vi "capstone1 ver 4_temp&move code.vi"() -> ()   [LabVIEW 2016]
uses:
  <instrlib>/Dynamixel Motor/Public/Motor Operation/Low Level/Baud Setting.ctl
  <vilib>/myRIO/Instrument Drivers/Onboard IO/DIO/typedefs/DIO Reference.ctl
  <vilib>/myRIO/Common/Instrument Driver Framework/Utilities/typedefs/myRIO Generic Hardware Reference.ctl
  <vilib>/myRIO/Common/Instrument Driver Framework/Utilities/typedefs/Hardware Version Enum.ctl
  <vilib>/myRIO/Common/Instrument Driver Framework/Utilities/typedefs/myRIO v1.0 Reference.ctl
  <vilib>/myRIO/Common/Instrument Driver Framework/Utilities/typedefs/Generic FPGA Reference.ctl
  <vilib>/myRIO/Common/Instrument Driver Framework/myRIO v1.0/DIO/typedefs/DIO Channels List.ctl
  <vilib>/myRIO/Common/Instrument Driver Framework/myRIO v1.0/DIO/typedefs/DIO Channels Enum.ctl
  <vilib>/userdefined/High Color/nirio_resource_hc.ctl
  <vilib>/myRIO/Common/Instrument Driver Framework/Utilities/vis/Is FPGA Ref Available.vi
  <vilib>/myRIO/Common/Instrument Driver Framework/myRIO v1.0/DIO/vis/myRIO v1.1 Open DIO.vi
  <vilib>/myRIO/Instrument Drivers/Onboard IO/DIO/vis/Write.vi
  <vilib>/myRIO/Common/Instrument Driver Framework/Utilities/vis/Validate Channels.vi
  <vilib>/myRIO/Common/Instrument Driver Framework/myRIO v1.0/DIO/vis/myRIO v1.0 Reserve DIO.vi
  <vilib>/myRIO/Common/Instrument Driver Framework/myRIO v1.0/Resource Manager/vis/myRIO v1.0 Reserve Channel List.vi
  <vilib>/myRIO/Common/Instrument Driver Framework/myRIO v1.0/DIO/vis/myRIO v1.0 Build MUX Configuration DIO.vi
  <vilib>/myRIO/Common/Instrument Driver Framework/myRIO v1.0/Resource Manager/vis/myRIO v1.0 Reserve Channel.vi
  <vilib>/myRIO/Common/Instrument Driver Framework/myRIO v1.0/Resource Manager/vis/myRIO v1.0 Unreserve Channel.vi
  <vilib>/myRIO/Common/Instrument Driver Framework/myRIO v1.0/Resource Manager/vis/myRIO v1.0 Create Configuration List.vi
  <vilib>/myRIO/Common/Instrument Driver Framework/myRIO v1.0/Resource Manager/vis/myRIO v1.0 Build Mutex Name.vi
  <vilib>/Utility/VariantDataType/GetNumericInfo.vi
  <vilib>/Utility/error.llb/Error Cluster From Error Code.vi
  <vilib>/myRIO/Common/Instrument Driver Framework/myRIO v1.0/myRIO v1.1 Open.vi
  <vilib>/myRIO/Common/Instrument Driver Framework/Utilities/vis/IO Manager.vi
  <vilib>/myRIO/Common/Instrument Driver Framework/Utilities/vis/Configuration Manager.vi
  <vilib>/myRIO/Common/Instrument Driver Framework/myRIO v1.0/Resource Manager/vis/myRIO v1.0 Configure IO.vi
  <vilib>/myRIO/Common/Instrument Driver Framework/myRIO v1.0/myRIO v1.0 Close.vi
  <vilib>/myRIO/Common/Instrument Driver Framework/myRIO v1.0/DIO/vis/myRIO v1.0 Write DIO.vi
  <vilib>/myRIO/Express VI/Onboard Devices/LED/LED Express VI.xnode
  <vilib>/myRIO/Instrument Drivers/Onboard IO/DIO/vis/myRIO DIO Open.xnode
  <instrlib>/Dynamixel Motor/Dynamixel Motor.lvlib
  <vilib>/myRIO/Instrument Drivers/Onboard IO/DIO/DIO.lvlib
panel:
  out "RT TCP Loop time 4":u32
  out "Numeric":i32
  out "RT TCP Loop time 3":u32
  out "RT TCP Loop time 2":u32
  out "RT TCP Loop time":u32
  out "motor temp":cluster{"0":sgl, "1":sgl, "2":sgl, "3":sgl}
  out "value":T1
  out "TCP Read data":string
  in  "정지":bool
  out "error out":errorcluster
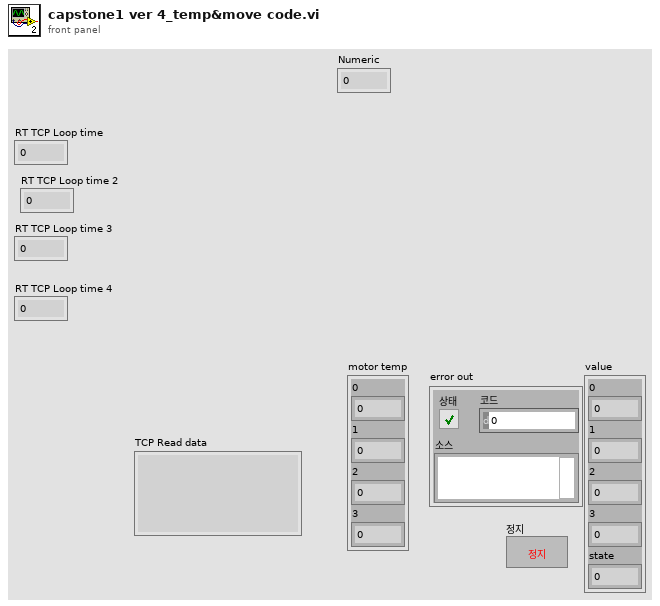
[diagram p1: front panel]
types:
  T1 = cluster{"0":sgl, "1":sgl, "2":sgl, "3":sgl, "state":sgl}
  T2 = typedef "Dynamixel Motor.lvlib/Baud Setting.ctl" = u8
  T3 = enum16{"big-endian, network order", "native, host order", "little-endian"}
  T4 = typedef "DIO.lvlib/DIO Reference.ctl" = cluster{"myRIO Reference":T5, "DIO Channels List":T9}
  T5 = typedef "myRIO Generic Hardware Reference.ctl" = cluster{"myRIO Model":T6, "myRIO Hardware Reference":T7}
  T6 = typedef "Hardware Version Enum.ctl" = enum16{"Unknown", "myRIO-1900", "myRIO-1950", "roboRIO", "NI ELVIS RIO CM"}
  T7 = typedef "myRIO v1.0 Reference.ctl" = cluster{"Generic FPGA Reference":T8, "Allow multiple opens":bool}
  T8 = typedef "Generic FPGA Reference.ctl" = refnum<k20>
  T9 = typedef "DIO Channels List.ctl" = T10[]
  T10 = typedef "DIO Channels Enum.ctl" = enum16{"Not Connected", "C/DIO0", "C/DIO1", "C/DIO2", "C/DIO3", "C/DIO4", "C/DIO5", "C/DIO6", "C/DIO7", "A/DIO0", "A/DIO1", "A/DIO2", "A/DIO3", "A/DIO4", "A/DIO5", "A/DIO6", "A/DIO7", "A/DIO8", "A/DIO9", "A/DIO10", "A/DIO11", "A/DIO12", "A/DIO13", "A/DIO14", "A/DIO15", "B/DIO0", "B/DIO1", "B/DIO2", "B/DIO3", "B/DIO4", "B/DIO5", "B/DIO6", "B/DIO7", "B/DIO8", "B/DIO9", "B/DIO10", "B/DIO11", "B/DIO12", "B/DIO13", "B/DIO14", "B/DIO15", "LED0", "LED1", "LED2", "LED3", "Button0", "DIO/DIO0", "DIO/DIO1", "DIO/DIO2", "DIO/DIO3", "DIO/DIO4", "DIO/DIO5", "DIO/DIO6", "DIO/DIO7", "DIO/DIO8", "DIO/DIO9", "SPI/CS0", "SPI/CS1", "SPI/CS2", "SPI/CS3", "LED RADIO (Green)", "LED RADIO (Red)", "LED COMM (Green)", "LED COMM (Red)", "LED MODE (Green)", "LED MODE (Red)"}
  T11 = typedef "nirio_resource_hc.ctl" = tag
  T12 = cluster{"0":sgl, "1":sgl, "2":sgl, "3":sgl, "state":i32}
  T13 = cluster{"Temperature (C)":u8, "Temperature (C)":u8, "Temperature (C)":u8, "Temperature (C)":u8}
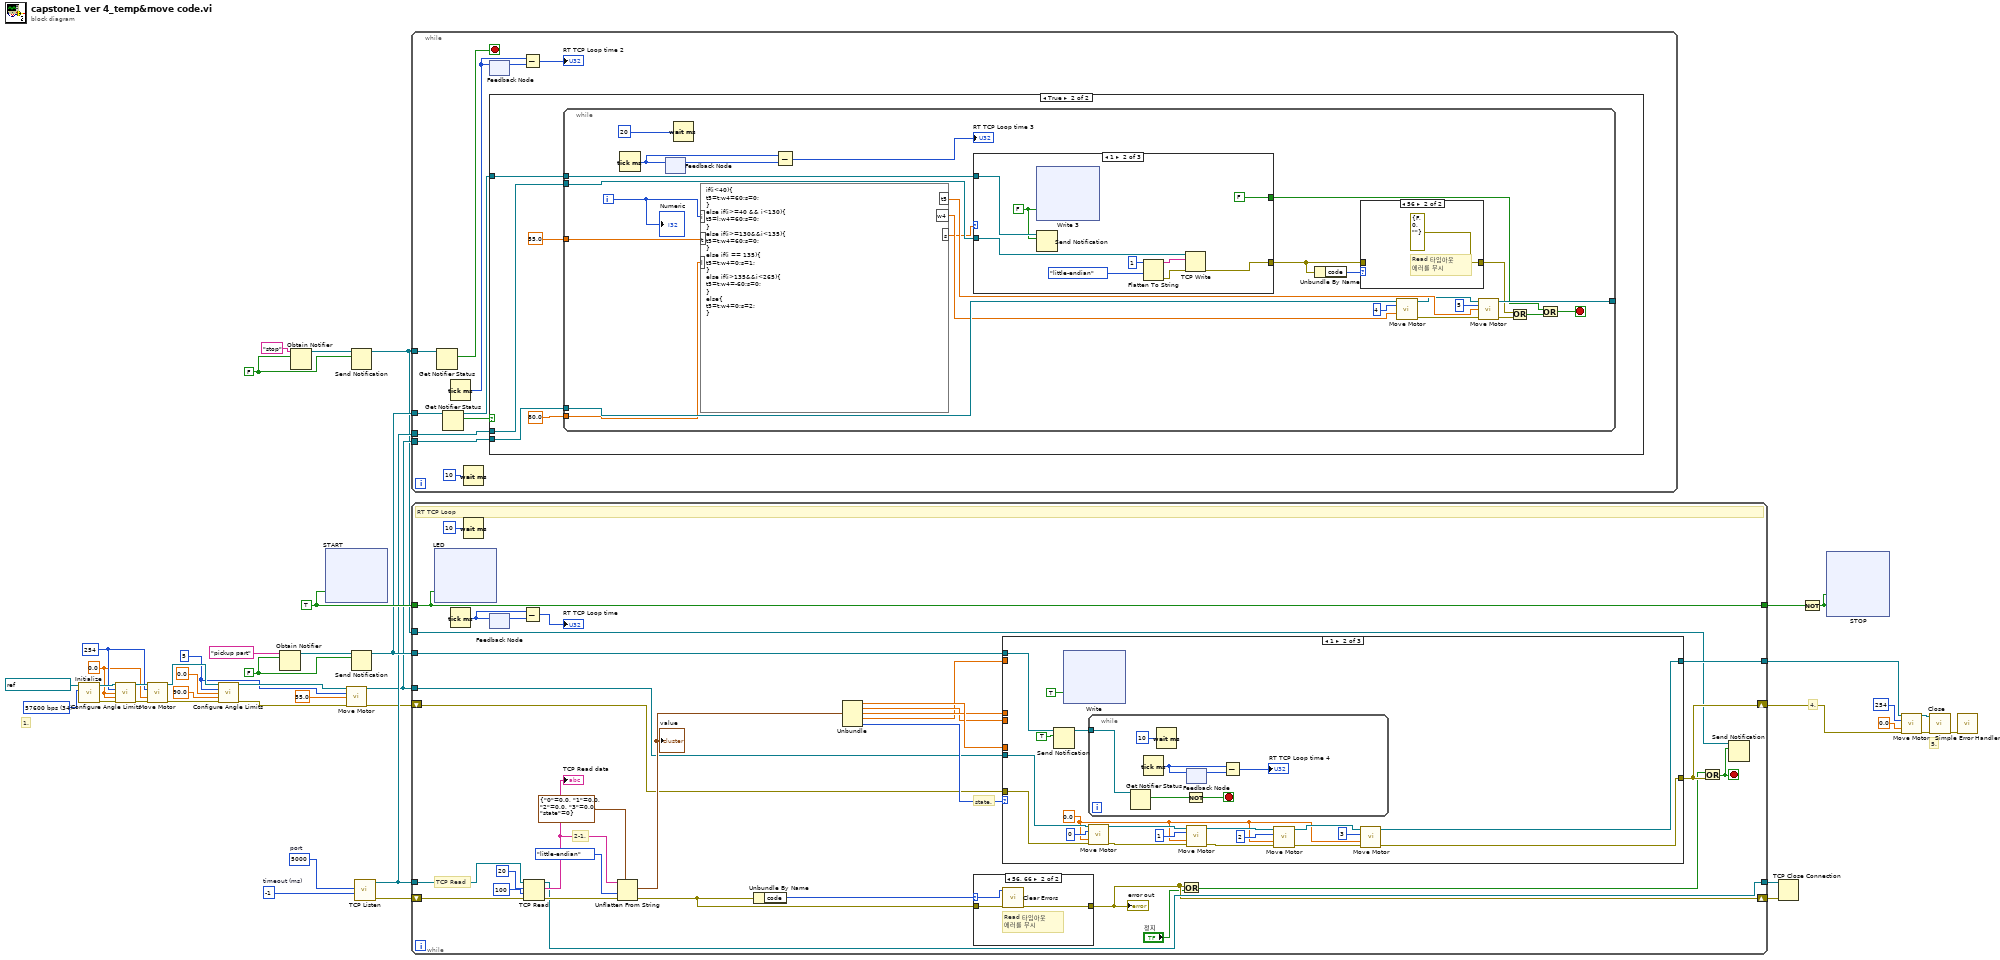
[diagram p0: block diagram]
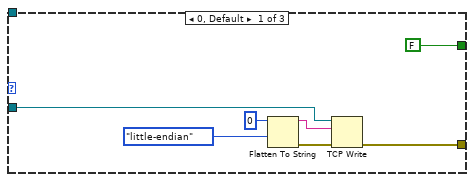
[diagram p4: hidden frame]
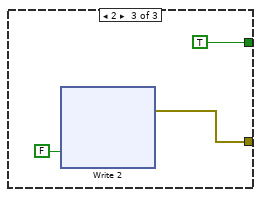
[diagram p5: hidden frame]
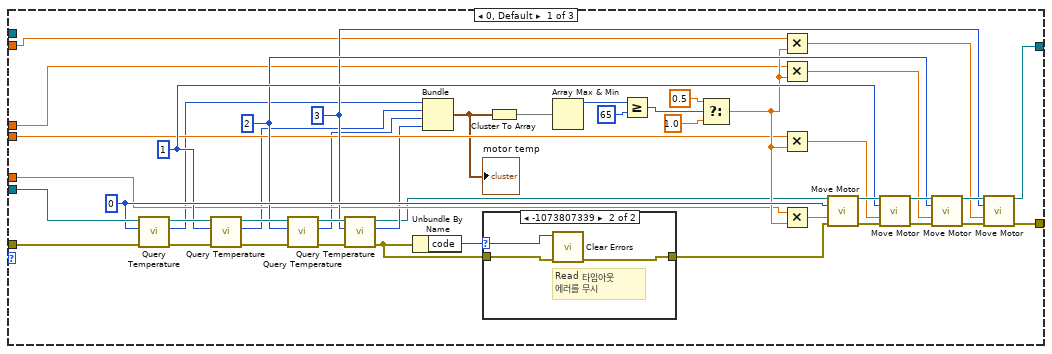
[diagram p6: hidden frame]
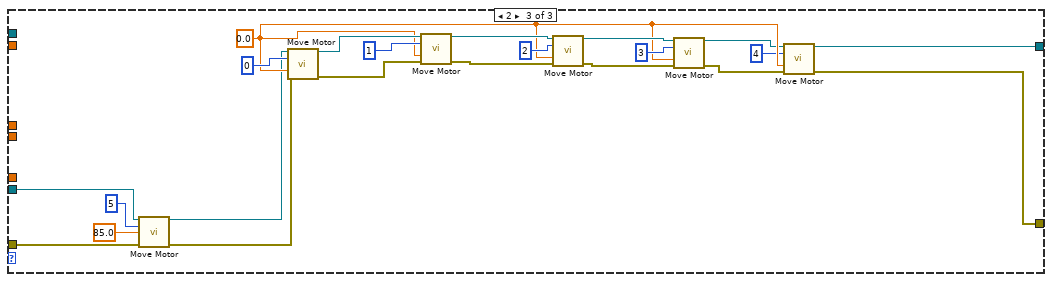
[diagram p8: hidden frame]
diagram:
  w3 = FALSE
  w14 = FALSE
  w6 = 5
  w37 = T2 34 items=["1,000,000 bps"=1, "500,000 bps"=3, "400,000 bps"=4, "250,000 bps"=7, "200,000 bps"=9, "115200 bps"=16, "57600 bps"=34, "19200 bps"=103, "9600 bps"=207] ("Baud rate (57600 bps)")
  w22 = TRUE
  w24 = u8 254 ("Motor ID (0)")
  w23 = 0.0 ("Clockwise Angle Limit (0 deg)")
  w41 = u16 5000  # port
  w42 = -1  # timeout (ms)
  # "5."
  # "4."
  # "1."
  n1 = call <instrlib>:"Initialize.vi"("Baud rate (57600 bps)"=w37, "VISA resource name"=refnum<visa-resource-name> "ASRL3::INSTR") -> ("error out"=w31:errorcluster, "VISA resource name out"=w30:refnum<visa-resource-name>)  [unwired: 8 in]
  n2 = call <instrlib>:"Configure Angle Limits.vi"("VISA resource name"=w30, "Motor ID (0)"=w24, "Clockwise Angle Limit (0 deg)"=w23, "Counter-Clockwise Angle Limit (300 deg)"=w23, "error in (no error)"=w31) -> ("VISA resource name out"=w26:refnum<visa-resource-name>, "error out"=w25:errorcluster)  [unwired: 9 in]
  n3 = call <instrlib>:"Move Motor.vi"("VISA resource name"=w26, "Motor ID (0)"=w24, "Goal Speed (RPM)"=w23, "error in (no error)"=w25) -> ("VISA resource name out"=w20:refnum<visa-resource-name>, "error out"=w21:errorcluster)  [unwired: 10 in]
  n4 = call <instrlib>:"Configure Angle Limits.vi"("VISA resource name"=w20, "Motor ID (0)"=w6, "Clockwise Angle Limit (0 deg)"=0.0, "Counter-Clockwise Angle Limit (300 deg)"=90.0 ("Clockwise Angle Limit (0 deg)"), "error in (no error)"=w21) -> ("VISA resource name out"=w10:refnum<visa-resource-name>, "error out"=w9:errorcluster)  [unwired: 9 in]
  n5 = Obtain Notifier(name (unnamed)="pickup part", notification data type=w14) -> (notifier out=w15:refnum<notifier>)  [unwired: 2 in, 2 out]
  n6 = Obtain Notifier(name (unnamed)="stop", notification data type=w3) -> (notifier out=w4:refnum<notifier>)  [unwired: 2 in, 2 out]
  n7 = xnode "START"("LED0"=w22) -> ()  [unwired: 1 in, 1 out]
  n8 = call <instrlib>:"Move Motor.vi"("VISA resource name"=w10, "Motor ID (0)"=w6, "Goal Position (180 deg)"=55.0, "error in (no error)"=w9) -> ("VISA resource name out"=w7:refnum<visa-resource-name>, "error out"=w8:errorcluster)  [unwired: 10 in]
  n9 = Send Notification(notification=w3, notifier=w4) -> (notifier out=w1:refnum<notifier>)  [unwired: 1 in, 1 out]
  n10 = Send Notification(notification=w14, notifier=w15) -> (notifier out=w13:refnum<notifier>)  [unwired: 1 in, 1 out]
  n11 = call <vilib>:"TCP Listen.vi"("timeout ms (wait forever: -1)"=w42, "port"=w41) -> ("error out"=w38:errorcluster, "connection ID"=w12:refnum<k5>)  [unwired: 5 in, 3 out]
  n12 = while {
    tunnel: w13 -> [w52]
    tunnel: w7 -> [w49]
    tunnel: w12 -> [w48]
    tunnel: w1 -> [w44]
    stop <- w43 stop-if-true
    n13 = Get Notifier Status(notifier=w44) -> (current notification=w43:bool)  [unwired: 1 in, 4 out]
    n14 = Get Notifier Status(notifier=w52) -> (notifier out=w50:refnum<notifier>, current notification=w51:bool)  [unwired: 1 in, 3 out]
    n15 = Tick Count (ms)() -> (millisecond timer value=w46:u32)
    n16 = Wait (ms)(milliseconds to wait=u32 10 ("대기 시간 (ms)")) -> ()  [unwired: 1 out]
    n17 = feedback #1() -> (w47:u32)  [unwired: 1 in]
    n18 = feedback-in #1(w46) -> ()
    n19 = case shown="True" w51 {
      tunnel: w50 -> [_ w54]
      tunnel: w49 -> [_ w58]
      tunnel: w48 -> [_ w57]
      frame False {
      }
      frame True {
        n20 = while {
          tunnel: w57 -> [w78]
          tunnel: w58 -> [w82]
          tunnel: [w77] -> _
          tunnel: 55.0 -> [w74]
          tunnel: 80.0 -> [w73]
          tunnel: w54 -> [w71]
          i -> [w80]
          stop <- w62 stop-if-true
          n21 = Tick Count (ms)() -> (millisecond timer value=w68:u32)
          n22 = feedback #2() -> (w69:u32)  [unwired: 1 in]
          n23 = feedback-in #2(w68) -> ()
          n24 = Wait (ms)(milliseconds to wait=u32 20 ("대기 시간 (ms)")) -> ()  [unwired: 1 out]
          n25 = formula code="if(i<40){\nt5=t;w4=60;s=0;\n}\nelse if(i>=40 && i<130){\nt5=l;w4=60;s=0;\n}\nelse if(i>=130&&i<135){\nt5=t;w4=60;s=0;\n}\nelse if(i == 135){\nt5=t;w4=0;s=1;\n}\nelse if(i>135&&i<265){\nt5=t;w4=-60;s=0;\n}\nelse{\nt5=t;w4=0;s=2;\n}"("i"=w80, "t"=w74, "l"=w73) -> ("t5"=w75:dbl, "w4"=w79:dbl, "s"=w70:dbl)
          n26 = Subtract(x=w68, y=w69) -> (x-y=→"RT TCP Loop time 3":u32)
          n27 = case shown="1" w70 {
            tunnel: w78 -> [w89 w101 _]
            tunnel: w71 -> [_ w97 _]
            tunnel: [FALSE FALSE TRUE] -> w64
            tunnel: [w86 w94 w137] -> w60
            frame 0, Default {
              n28 = Flatten To String(anything=0, byte order (0:big-endian, network order)=T3."little-endian") -> (data string=w90:string, error out=w87:errorcluster)  [unwired: 2 in, 1 out]
              n29 = TCP Write(connection ID=w89, data in=w90, error in (no error)=w87) -> (error out=w86:errorcluster)  [unwired: 1 in, 2 out]
            }
            frame 1 {
              w93 = FALSE ("notification")
              n30 = xnode "Write 3"("LED2"=w93) -> ()  [unwired: 1 in, 1 out]
              n31 = Send Notification(notification=w93, notifier=w97) -> ()  [unwired: 1 in, 2 out]
              n32 = Flatten To String(anything=1, byte order (0:big-endian, network order)=T3."little-endian") -> (data string=w98:string, error out=w95:errorcluster)  [unwired: 2 in, 1 out]
              n33 = TCP Write(connection ID=w101, data in=w98, error in (no error)=w95) -> (error out=w94:errorcluster)  [unwired: 1 in, 2 out]
            }
            frame 2 {
              n34 = xnode "Write 2"("LED2"=FALSE) -> ("error out"=w137:errorcluster)  [unwired: 1 in]
            }
          }
          n35 = Unbundle By Name(w60) -> ("code"=w61:i32)
          n36 = case shown="56" w61 {
            tunnel: [w84 errorcluster {"status"=FALSE, "code"=0, "source"=""} ("에러 출력")] -> w59
            tunnel: w60 -> [w84 _]
            frame 0, Default {
            }
            frame 56 {
              # "Read 타임아웃\n에러를 무시"
            }
          }
          n37 = call <instrlib>:"Move Motor.vi"("VISA resource name"=w82, "Motor ID (0)"=4, "Goal Speed (RPM)"=w79) -> ("VISA resource name out"=w72:refnum<visa-resource-name>, "error out"=w66:errorcluster)  [unwired: 11 in]
          n38 = call <instrlib>:"Move Motor.vi"("VISA resource name"=w72, "Motor ID (0)"=5, "Goal Position (180 deg)"=w75, "error in (no error)"=w66) -> ("VISA resource name out"=w77:refnum<visa-resource-name>, "error out"=w65:errorcluster)  [unwired: 10 in]
          n39 = Or(x=w59, y=w65) -> (x .or. y?=w63:bool)
          n40 = Or(x=w64, y=w63) -> (x .or. y?=w62:bool)
          "Numeric" <- w80
        }
      }
    }
    n41 = Subtract(x=w46, y=w47) -> (x-y=→"RT TCP Loop time 2":u32)
  }
  n42 = while {
    tunnel: w12 -> [w196]
    tunnel: [w180] -> w40
    shift-right: [w179] -> w39
    shift-left: w38 -> [w197]
    shift-right: [w186] -> w19
    shift-left: w8 -> [w185]
    tunnel: w22 -> [w195]
    tunnel: [w195] -> w33
    tunnel: w7 -> [w188]
    tunnel: [w187] -> w18
    tunnel: w13 -> [w178]
    tunnel: w1 -> [w176]
    stop <- w175 stop-if-true
    # "state."
    # "2-1."
    # "TCP Read"
    # "RT TCP Loop"
    n43 = xnode "LED"("LED1"=w195) -> ()  [unwired: 1 in, 1 out]
    n44 = Tick Count (ms)() -> (millisecond timer value=w182:u32)
    n45 = Wait (ms)(milliseconds to wait=u32 10 ("대기 시간 (ms)")) -> ()  [unwired: 1 out]
    n46 = feedback #3() -> (w183:u32)  [unwired: 1 in]
    n47 = feedback-in #3(w182) -> ()
    n48 = Subtract(x=w182, y=w183) -> (x-y=→"RT TCP Loop time":u32)
    n49 = TCP Read(connection ID=w196, bytes to read=20 ("읽을 바이트"), error in (no error)=w197, 9:100 ("타임아웃 ms (25000)")) -> (connection ID out=w180:refnum<k5>, data out=w200:string, error out=w199:errorcluster)  [unwired: 1 in]
    "TCP Read data" <- w200
    n50 = Unflatten From String(type=T12 {"0"=0.0, "1"=0.0, "2"=0.0, "3"=0.0, "state"=0}, binary string=w200, byte order (0:big-endian, network order)=T3."little-endian", error in (no error)=w199) -> (value=w194:T12, error out=w198:errorcluster)  [unwired: 1 in, 1 out]
    "value" <- w194
    n51 = Unbundle By Name(w198) -> ("code"=w205:i32)
    n52 = Unbundle(w194) -> ("0"=w193:sgl, "1"=w191:sgl, "2"=w192:sgl, "3"=w190:sgl, "state"=w189:i32)
    n53 = case shown="56, 66" w205 {
      selector: w205 -> [_ w375]
      tunnel: [w373 w374] -> w179
      tunnel: w198 -> [w373 w376]
      frame 0, Default {
      }
      frame 56, 66 {
        # "Read 타임아웃\n에러를 무시"
        n54 = call <vilib>:"Clear Errors.vi"("error in (no error)"=w376, "specific error code to clear (0: all)"=w375) -> ("error out"=w374:errorcluster)  [unwired: 4 in, 1 out]
      }
    }
    "error out" <- w179
    n55 = case shown="1" w189 {
      tunnel: w193 -> [w229 _ _]
      tunnel: w191 -> [w227 _ _]
      tunnel: w192 -> [w225 _ _]
      tunnel: w190 -> [w223 _ _]
      tunnel: w188 -> [w241 w263 w318]
      tunnel: [w211 w260 w324] -> w187
      tunnel: [w212 w259 w323] -> w186
      tunnel: w185 -> [w213 w261 w320]
      tunnel: w178 -> [_ w258 _]
      frame 0, Default {
        w237 = 3
        w238 = 2
        w239 = 1
        w240 = 0
        n56 = call <instrlib>:"Query Temperature.vi"("error in"=w213, "Motor ID (0)"=w240, "VISA resource name"=w241) -> ("error out"=w236:errorcluster, "Temperature (C)"=w221:u8, "VISA resource name out"=w244:refnum<visa-resource-name>)  [unwired: 6 in]
        n57 = call <instrlib>:"Query Temperature.vi"("error in"=w236, "Motor ID (0)"=w239, "VISA resource name"=w244) -> ("error out"=w235:errorcluster, "Temperature (C)"=w220:u8, "VISA resource name out"=w243:refnum<visa-resource-name>)  [unwired: 6 in]
        n58 = call <instrlib>:"Query Temperature.vi"("error in"=w235, "Motor ID (0)"=w238, "VISA resource name"=w243) -> ("error out"=w234:errorcluster, "Temperature (C)"=w219:u8, "VISA resource name out"=w242:refnum<visa-resource-name>)  [unwired: 6 in]
        n59 = call <instrlib>:"Query Temperature.vi"("error in"=w234, "Motor ID (0)"=w237, "VISA resource name"=w242) -> ("error out"=w208:errorcluster, "Temperature (C)"=w218:u8, "VISA resource name out"=w210:refnum<visa-resource-name>)  [unwired: 6 in]
        n60 = Unbundle By Name(w208) -> ("code"=w209:i32)
        n61 = Bundle("Temperature (C)"=w221, "Temperature (C)"=w220, "Temperature (C)"=w219, "Temperature (C)"=w218) -> (w215:T13)  [unwired: 1 in]
        "motor temp" <- w215
        n62 = case shown="-1073807339" w209 {
          selector: w209 -> [_ w253]
          tunnel: [w251 w252] -> w207
          tunnel: w208 -> [w251 w254]
          frame 0, Default {
          }
          frame -1073807339 {
            # "Read 타임아웃\n에러를 무시"
            n63 = call <vilib>:"Clear Errors.vi"("error in (no error)"=w254, "specific error code to clear (0: all)"=w253) -> ("error out"=w252:errorcluster)  [unwired: 4 in, 1 out]
          }
        }
        n64 = Cluster To Array(cluster=w215) -> (array=w217:u8[])
        n65 = Array Max & Min(array=w217) -> (max value=w216:u8)  [unwired: 3 out]
        n66 = Greater Or Equal?(x=w216, y=65) -> (x >= y?=w214:bool)
        n67 = Select(t=0.5, s=w214, f=1.0) -> (s? t:f=w230:dbl)
        n68 = Multiply(x=w223, y=w230) -> (x*y=w222:dbl)
        n69 = Multiply(x=w225, y=w230) -> (x*y=w224:dbl)
        n70 = Multiply(x=w227, y=w230) -> (x*y=w226:dbl)
        n71 = Multiply(x=w229, y=w230) -> (x*y=w228:dbl)
        n72 = call <instrlib>:"Move Motor.vi"("VISA resource name"=w210, "Motor ID (0)"=w240, "Goal Speed (RPM)"=w228, "error in (no error)"=w207) -> ("VISA resource name out"=w245:refnum<visa-resource-name>, "error out"=w246:errorcluster)  [unwired: 10 in]
        n73 = call <instrlib>:"Move Motor.vi"("VISA resource name"=w245, "Motor ID (0)"=w239, "Goal Speed (RPM)"=w226, "error in (no error)"=w246) -> ("VISA resource name out"=w247:refnum<visa-resource-name>, "error out"=w249:errorcluster)  [unwired: 10 in]
        n74 = call <instrlib>:"Move Motor.vi"("VISA resource name"=w247, "Motor ID (0)"=w238, "Goal Speed (RPM)"=w224, "error in (no error)"=w249) -> ("VISA resource name out"=w248:refnum<visa-resource-name>, "error out"=w250:errorcluster)  [unwired: 10 in]
        n75 = call <instrlib>:"Move Motor.vi"("VISA resource name"=w248, "Motor ID (0)"=w237, "Goal Speed (RPM)"=w222, "error in (no error)"=w250) -> ("VISA resource name out"=w211:refnum<visa-resource-name>, "error out"=w212:errorcluster)  [unwired: 10 in]
      }
      frame 1 {
        w262 = 0.0
        n76 = Send Notification(notification=TRUE, notifier=w258) -> (notifier out=w256:refnum<notifier>)  [unwired: 1 in, 1 out]
        n77 = xnode "Write"("LED2"=TRUE) -> ()  [unwired: 1 in, 1 out]
        n78 = while {
          tunnel: w256 -> [w314]
          stop <- w312 stop-if-true
          n79 = Get Notifier Status(notifier=w314) -> (current notification=w313:bool)  [unwired: 1 in, 4 out]
          n80 = Tick Count (ms)() -> (millisecond timer value=w309:u32)
          n81 = Wait (ms)(milliseconds to wait=u32 10 ("대기 시간 (ms)")) -> ()  [unwired: 1 out]
          n82 = Not(x=w313) -> (.not. x?=w312:bool)
          n83 = feedback #4() -> (w311:u32)  [unwired: 1 in]
          n84 = feedback-in #4(w309) -> ()
          n85 = Subtract(x=w309, y=w311) -> (x-y=→"RT TCP Loop time 4":u32)
        }
        n86 = call <instrlib>:"Move Motor.vi"("VISA resource name"=w263, "Motor ID (0)"=0, "Goal Speed (RPM)"=w262, "error in (no error)"=w261) -> ("VISA resource name out"=w264:refnum<visa-resource-name>, "error out"=w265:errorcluster)  [unwired: 10 in]
        n87 = call <instrlib>:"Move Motor.vi"("VISA resource name"=w264, "Motor ID (0)"=1, "Goal Speed (RPM)"=w262, "error in (no error)"=w265) -> ("VISA resource name out"=w266:refnum<visa-resource-name>, "error out"=w268:errorcluster)  [unwired: 10 in]
        n88 = call <instrlib>:"Move Motor.vi"("VISA resource name"=w266, "Motor ID (0)"=2, "Goal Speed (RPM)"=w262, "error in (no error)"=w268) -> ("VISA resource name out"=w267:refnum<visa-resource-name>, "error out"=w269:errorcluster)  [unwired: 10 in]
        n89 = call <instrlib>:"Move Motor.vi"("VISA resource name"=w267, "Motor ID (0)"=3, "Goal Speed (RPM)"=w262, "error in (no error)"=w269) -> ("VISA resource name out"=w260:refnum<visa-resource-name>, "error out"=w259:errorcluster)  [unwired: 10 in]
      }
      frame 2 {
        w327 = 0.0
        n90 = call <instrlib>:"Move Motor.vi"("VISA resource name"=w318, "Motor ID (0)"=5, "Goal Position (180 deg)"=85.0, "error in (no error)"=w320) -> ("VISA resource name out"=w317:refnum<visa-resource-name>, "error out"=w319:errorcluster)  [unwired: 10 in]
        n91 = call <instrlib>:"Move Motor.vi"("VISA resource name"=w317, "Motor ID (0)"=0, "Goal Speed (RPM)"=w327, "error in (no error)"=w319) -> ("VISA resource name out"=w337:refnum<visa-resource-name>, "error out"=w336:errorcluster)  [unwired: 10 in]
        n92 = call <instrlib>:"Move Motor.vi"("VISA resource name"=w337, "Motor ID (0)"=1, "Goal Speed (RPM)"=w327, "error in (no error)"=w336) -> ("VISA resource name out"=w335:refnum<visa-resource-name>, "error out"=w333:errorcluster)  [unwired: 10 in]
        n93 = call <instrlib>:"Move Motor.vi"("VISA resource name"=w335, "Motor ID (0)"=2, "Goal Speed (RPM)"=w327, "error in (no error)"=w333) -> ("VISA resource name out"=w334:refnum<visa-resource-name>, "error out"=w332:errorcluster)  [unwired: 10 in]
        n94 = call <instrlib>:"Move Motor.vi"("VISA resource name"=w334, "Motor ID (0)"=3, "Goal Speed (RPM)"=w327, "error in (no error)"=w332) -> ("VISA resource name out"=w325:refnum<visa-resource-name>, "error out"=w322:errorcluster)  [unwired: 10 in]
        n95 = call <instrlib>:"Move Motor.vi"("VISA resource name"=w325, "Motor ID (0)"=4, "Goal Speed (RPM)"=w327, "error in (no error)"=w322) -> ("VISA resource name out"=w324:refnum<visa-resource-name>, "error out"=w323:errorcluster)  [unwired: 10 in]
      }
    }
    n96 = Or(x=w179, y="정지") -> (x .or. y?=w184:bool)
    n97 = Or(x=w184, y=w186) -> (x .or. y?=w175:bool)
    n98 = Send Notification(notification=w175, notifier=w176) -> ()  [unwired: 1 in, 2 out]
  }
  n99 = TCP Close Connection(connection ID=w40, error in (no error)=w39) -> ()  [unwired: 3 out]
  n100 = Not(x=w33) -> (.not. x?=w32:bool)
  n101 = xnode "STOP"("LED0"=w32, "LED1"=w32) -> ()  [unwired: 1 in, 1 out]
  n102 = call <instrlib>:"Move Motor.vi"("VISA resource name"=w18, "Motor ID (0)"=u8 254, "Goal Speed (RPM)"=0.0, "error in (no error)"=w19) -> ("VISA resource name out"=w17:refnum<visa-resource-name>, "error out"=w16:errorcluster)  [unwired: 10 in]
  n103 = call <instrlib>:"Close.vi"("error in (no error)"=w16, "VISA resource name"=w17) -> ("error out"=w27:errorcluster)  [unwired: 9 in]
  n104 = call <vilib>:"Simple Error Handler.vi"("error in (no error)"=w27) -> ()  [unwired: 4 in, 5 out]
